vi "PH_Sound.PC _CountdownRunning.vi"(0 "i ref in":refnum<vi>, 3 "State CR":bool, 5 "error in (no error)":errorcluster) -> (14 "i ref out":refnum<vi>, 19 "error out":errorcluster)   [LabVIEW 2014, in "PH_Sound.lvlib"]
doc: "This VI writes the incoming countdown running state to own attributes and the GUI element."
uses:
  PH_Sound.lvlib
  PH_Common/PH_Common.lvlib
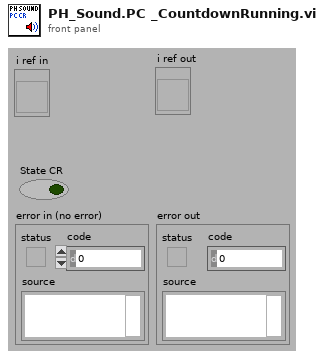
[diagram p1: front panel]
types:
  T1 = typedef "PH_Sound.lvlib/PH_Sound.i attribute.ctl" = cluster{"GUI Refs":cluster{"Exit":refnum<vi>, "Laserfreigabe":refnum<vi>, "PreAmp-Freigabe":refnum<vi>, "Countdown Running":refnum<vi>, "Emergency Off":refnum<vi>, "Device Error":refnum<vi>}, "Testalarm on":bool, "State":cluster{"Laser Class 4":bool, "PreAmp Running":bool, "Countdown Running":bool, "Emergency Off":bool}, "Starting Time":timestamp}
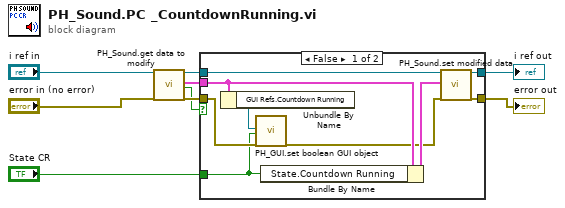
[diagram p0: block diagram]
diagram:
  n1 = call "PH_Sound.get data to modify.vi"("i ref in"="i ref in", "error in (no error)"="error in (no error)") -> ("i ref out"=w3:refnum<vi>, "i attribute"=w2:T1, "timed out"=w1:bool, "error out"=w4:errorcluster)  [unwired: 14 in]
  n2 = case shown="False" w1 {
    tunnel: w4 -> [w13 w19]
    tunnel: w3 -> [w16 w20]
    tunnel: [w18 w20] -> w7
    tunnel: [w17 w19] -> w6
    tunnel: w2 -> [w14 _]
    tunnel: "State CR" -> [w10 _]
    frame False {
      n3 = Unbundle By Name(w14) -> ("GUI Refs.Countdown Running"=w11:refnum<vi>)
      n4 = call "PH_GUI.set boolean GUI object.vi"("Boolean Knob GUI Ref"=w11, "Value"=w10, "error in (no error)"=w13) -> ("error out"=w12:errorcluster)  [unwired: 16 in]
      n5 = Bundle By Name(cluster=w14, "State.Countdown Running"=w10) -> (w15:T1)
      n6 = call "PH_Sound.set modified data.vi"("i ref in"=w16, "i attribute"=w15, "error in (no error)"=w12) -> ("i ref out"=w18:refnum<vi>, "error out"=w17:errorcluster)  [unwired: 15 in]
    }
    frame True {
    }
  }
  "error out" <- w6
  "i ref out" <- w7
